vi "getStatusMovingAllAxes.vi"(0 "connection ID":refnum<k5>, 5 "error in":errorcluster) -> (14 "connection ID":refnum<k5>, 15 "moving1":i32, 16 "moving2":i32, 17 "moving3":i32, 19 "error out":errorcluster)   [LabVIEW 2016, in "AMC_VIs.lvlib"]
doc: "Get Status of all axes, see getStatusMoving for coding of the values"
uses:
  AMC_VIs.lvlib
panel:
  out "params_cluster":cluster{"Numeric":i32}
  in  "Params_cluster":cluster{"Numeric":dbl}
  in  "results_cluster":T1
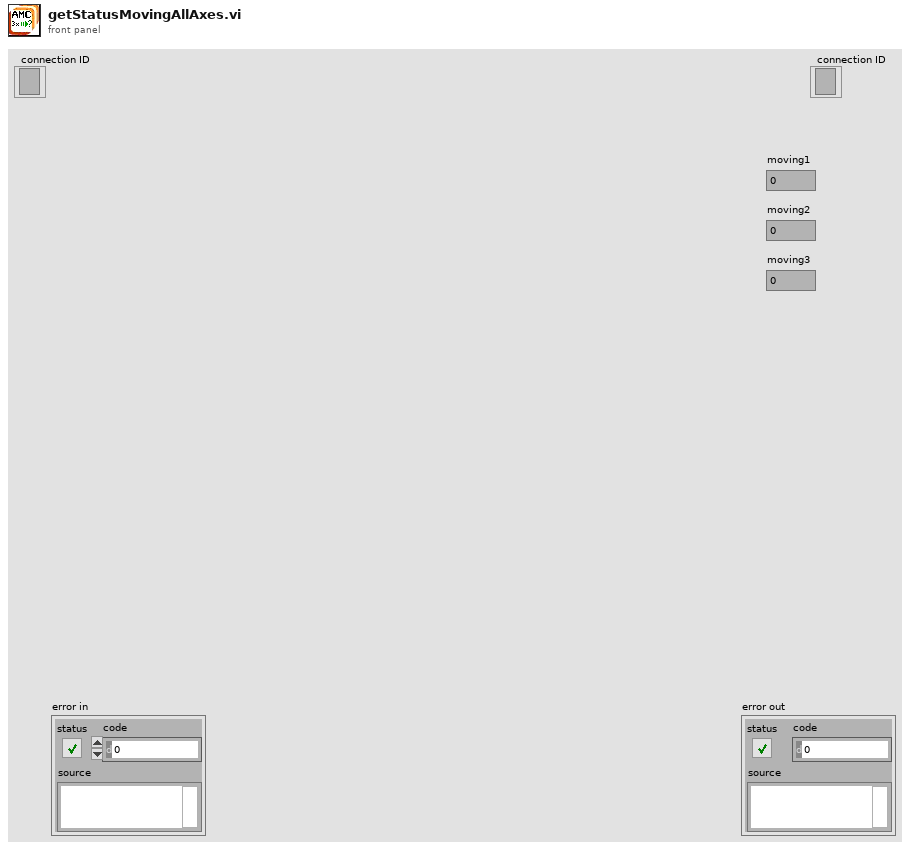
[diagram p1: front panel]
types:
  T1 = cluster{"errNo":i32, "moving1":i32, "moving2":i32, "moving3":i32}
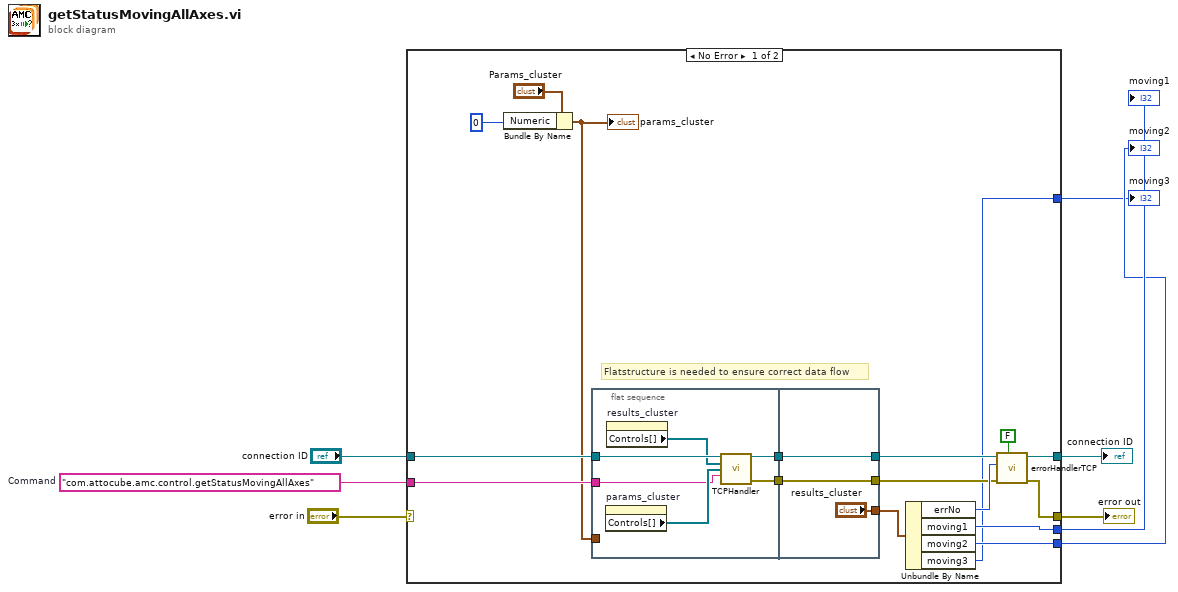
[diagram p0: block diagram]
diagram:
  w4 = "com.attocube.amc.control.getStatusMovingAllAxes"  # Command
  n1 = case shown="No Error" "error in" {
    selector: "error in" -> [_ w36]
    tunnel: [w23 w36] -> w8
    tunnel: [w25 w35] -> w7
    tunnel: "connection ID" -> [w22 w35]
    tunnel: w4 -> [w16 _]
    tunnel: [w11 _] -> w3
    tunnel: [w10 _] -> w2
    tunnel: [w9 _] -> w1
    frame No Error {
      # "Flatstructure is needed to ensure correct data flow"
      n2 = Bundle By Name(cluster="Params_cluster", "Numeric"=0) -> (w13:cluster{"Numeric":dbl})
      "params_cluster" <- w13
      n3 = flat-sequence {
        tunnel: [w30] -> w18
        tunnel: w22 -> [w31]
        tunnel: w16 -> [w27]
        tunnel: [w26] -> w14
        tunnel: w13 -> [_]
        tunnel: ["results_cluster"] -> w19
        tunnel: [w34] -> w21
        tunnel: w18 -> [w34]
        tunnel: [w32] -> w15
        tunnel: w14 -> [w32]
        frame #0 {
          n4 = property on="params_cluster" class="Clust (strict)"() -> ("Controls[]"=w28:refnum<vi>[])  [unwired: 2 in, 2 out]
          n5 = property on="results_cluster" class="Clust (strict)"() -> ("Controls[]"=w29:refnum<vi>[])  [unwired: 2 in, 2 out]
          n6 = call "TCPHandler.vi"("connection ID"=w31, "results_cluster"=w29, "params_cluster"=w28, "method"=w27) -> ("connection ID"=w30:refnum<k5>, "error"=w26:errorcluster)  [unwired: 8 in, 2 out]
        }
        frame #1 {
        }
      }
      n7 = Unbundle By Name(w19) -> ("errNo"=w20:i32, "moving1"=w11:i32, "moving2"=w10:i32, "moving3"=w9:i32)
      n8 = call "errorHandlerTCP.vi"("show popup"=FALSE, "error in"=w15, "error number"=w20, "connection ID"=w21) -> ("error out"=w23:errorcluster, "connection ID"=w25:refnum<k5>)  [unwired: 6 in]
    }
    frame Error {
    }
  }
  "error out" <- w8
  "connection ID" <- w7
  "moving1" <- w3
  "moving2" <- w2
  "moving3" <- w1
